vi "Get visa 1d DBL data.vi"(7 "VISA resource name":refnum<visa-resource-name>, 8 "error in (no error)":errorcluster, 9 "Name":string, 10 "Mag Lab Parameters in":refnum<class "Mag Lab Parameters.lvclass">, 11 "AH 2500 in":refnum<class "AH 2500.lvclass">) -> (0 "error out":errorcluster, 1 "Channel data":dbl[](array[numeric]), 2 "Channel names":string[](array[string]), 3 "AH 2500 out":refnum<class "AH 2500.lvclass">, 5 "VISA resource name out":refnum<visa-resource-name>)   [LabVIEW 2015, in "AH 2500.lvclass"]
uses:
  AH 2500.lvclass
  Mag Lab Properties/Mag Lab Parameters.lvclass
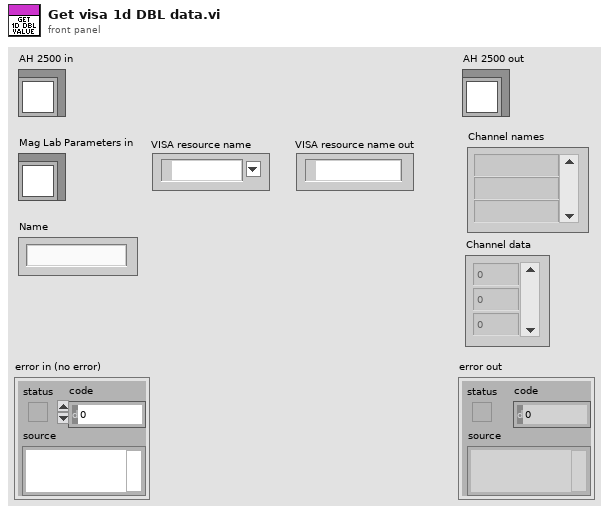
[diagram p1: front panel]
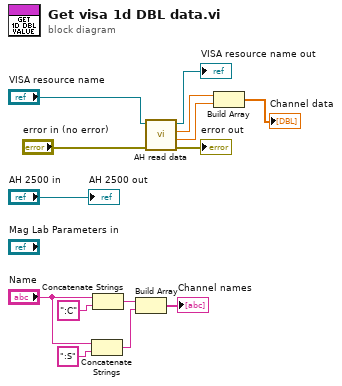
[diagram p0: block diagram]
diagram:
  n1 = Concatenate Strings("Name", ":S" ("string")) -> (w9:string)
  n2 = Concatenate Strings("Name", ":C" ("string")) -> (w11:string)
  n3 = Build Array(w11, w9) -> (→"Channel names":string[])
  n4 = call "AH read data.vi"("error in (no error)"="error in (no error)", "VISA Resource Name"="VISA resource name") -> ("error out"=→"error out":errorcluster, "Loss"=w1:dbl, "Capacitance"=w2:dbl, "VISA Resource Name Out"=→"VISA resource name out":refnum<visa-resource-name>)  [unwired: 6 in]
  n5 = Build Array(w2, w1) -> (→"Channel data":dbl[])
  "AH 2500 out" <- "AH 2500 in"
